vi "NI9188 Producer (Testing).vi"(5 "TDMS File Path":path, 7 "Logging Mode":i32(ring)=10231 items=["Off"=10231, "Log and Read"=15842], 8 "error in":errorcluster, 9 "Samples per Channel":i32=100, 10 "Sample Rate":dbl=100000.0, 11 "Data Queue":refnum<queue>) -> (0 "error out":errorcluster, 2 "Restart":bool)   [LabVIEW 2013]
uses:
  <vilib>/DAQmx/create/channels.llb/DAQmx Create Channel (AI-Voltage-Basic).vi
  <vilib>/DAQmx/configure/timing.llb/DAQmx Timing (Sample Clock).vi
  <vilib>/DAQmx/configure/task.llb/DAQmx Configure Logging (TDMS).vi
  <vilib>/DAQmx/create/channels.llb/DAQmx Create Channel (CO-Pulse Generation-Frequency).vi
  <vilib>/DAQmx/configure/timing.llb/DAQmx Timing (Implicit).vi
  <vilib>/DAQmx/configure/trigger.llb/DAQmx Start Trigger (Digital Edge).vi
  SCM Breakdown Locator/UDP Heartbeat Globals.vi
  Execution Control Global.vi
  <vilib>/DAQmx/read.llb/DAQmx Read (Analog 1D Wfm NChan NSamp).vi
  <resource>/objmgr/daqmx.rc
panel:
  out "name":string
  in  "Remote UDP Port":u16=31416
  out "Spark Flag Synch\nLoop Time (ms)":u32
  in  "Stop":bool
  out "Spark!":bool
  in  "Local UDP Port":u16=31417
  in  "Synch Delay (ms)":u16=50
  out "ms since last read":u32
  out "Waveform Graph":waveform(dbl)[](graph)
  out "Actual Sample Rate":dbl=1000.0 format="%0.2f"
  # "Acquired Data"
  # "Settings"
  # "Logging Settings"
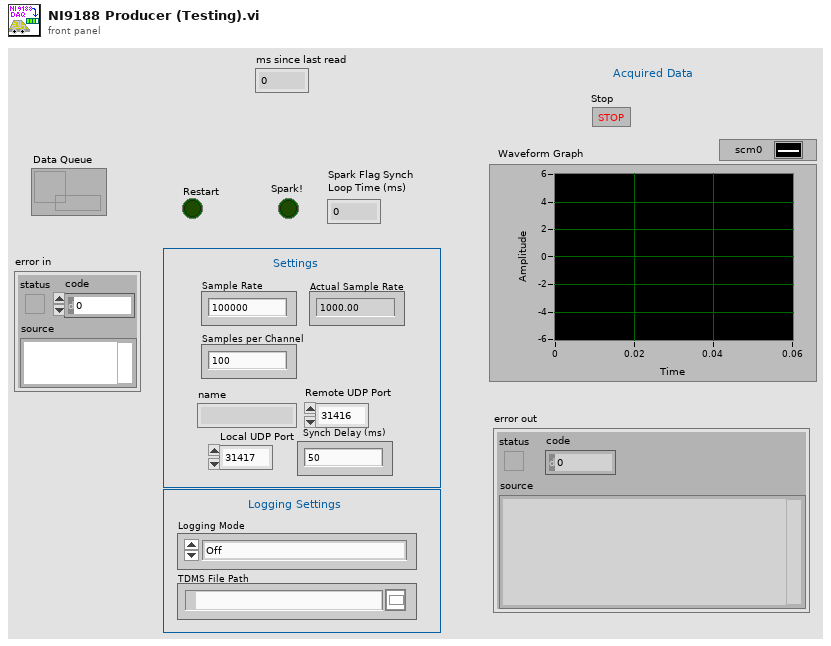
[diagram p1: front panel]
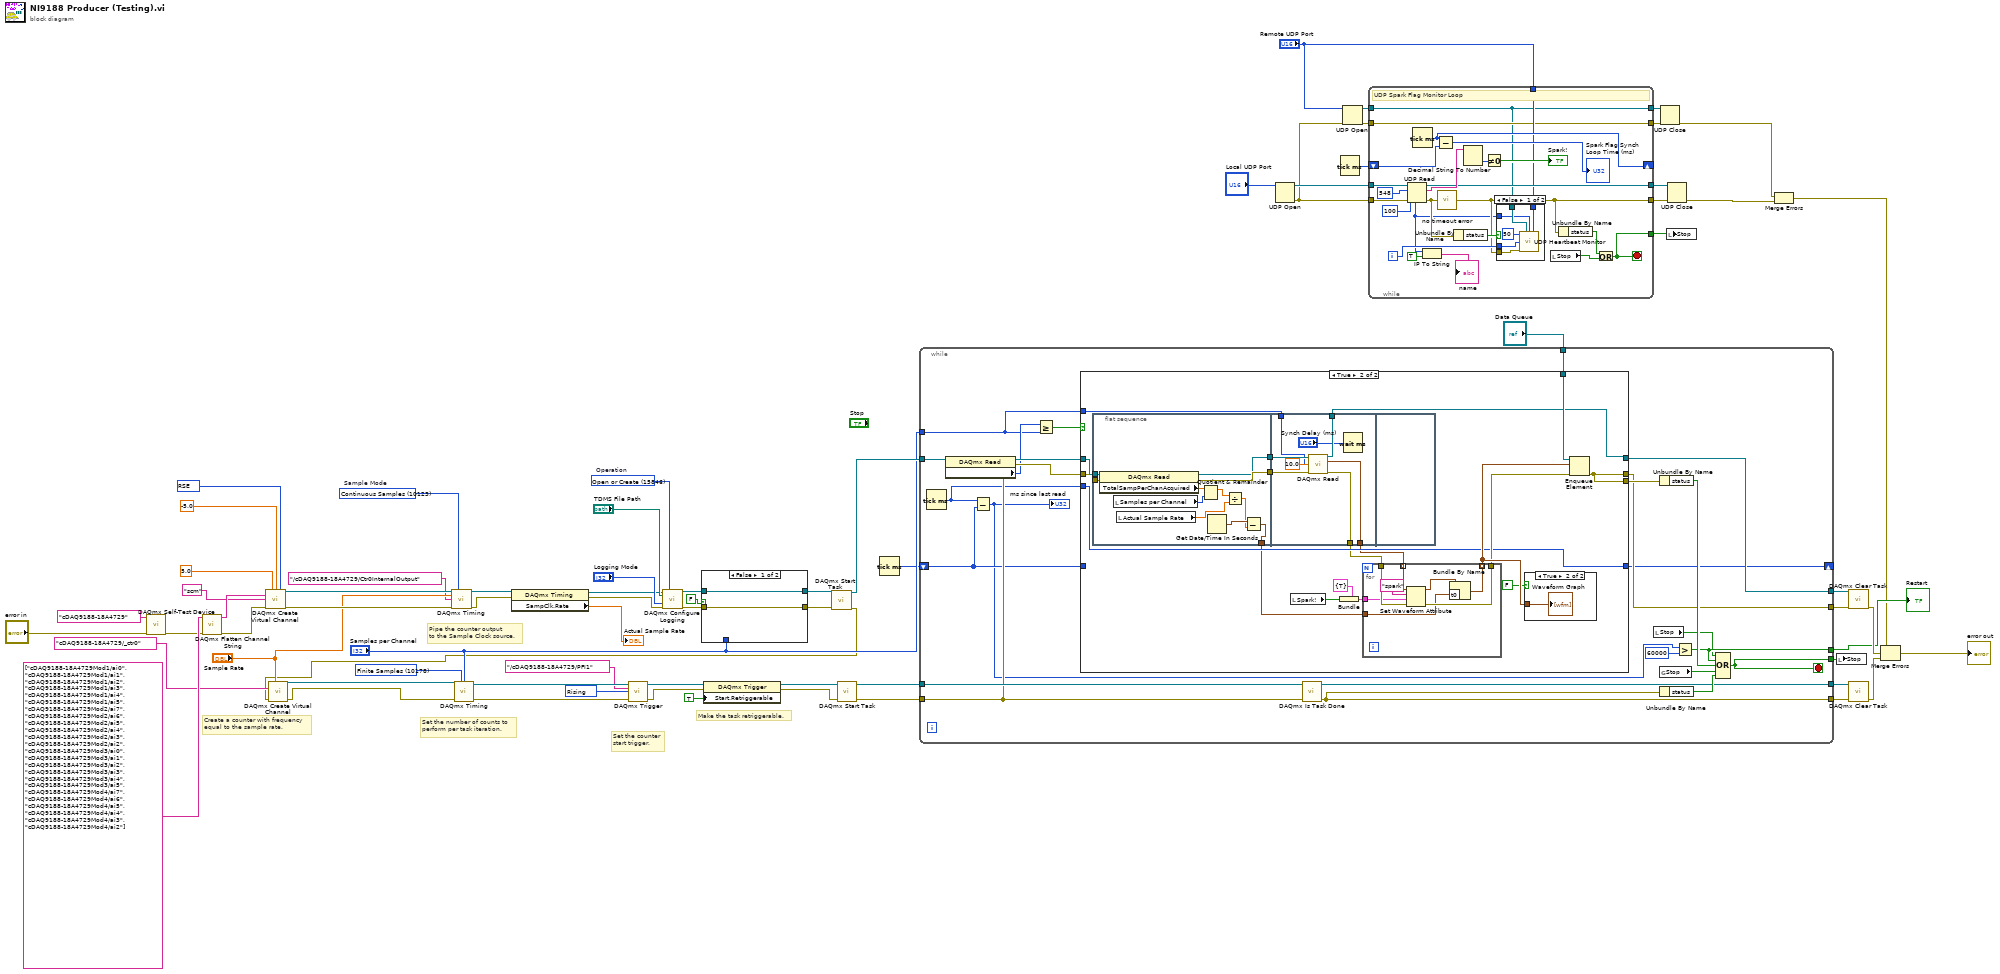
[diagram p0: block diagram]
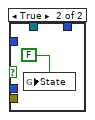
[diagram p2: hidden frame]
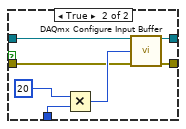
[diagram p3: hidden frame]
diagram:
  w30 = 10280 items=["Rising"=10280, "Falling"=10171] ("edge")
  w64 = 10083 items=["default"=-1, "RSE"=10083, "NRSE"=10078, "Differential"=10106, "Pseudodifferential"=12529] ("Terminal Configuration")
  w54 = 10178 items=["Finite Samples"=10178, "Continuous Samples"=10123, "Hardware Timed Single Point"=12522] ("sample mode")
  w67 = 15846 items=["Open"=10437, "Open or Create"=15846, "Create or Replace"=15847, "Create"=15848]  # Operation
  w70 = 10123 items=["Finite Samples"=10178, "Continuous Samples"=10123, "Hardware Timed Single Point"=12522]  # Sample Mode
  # "Set the counter\nstart trigger."
  # "Make the task retriggerable."
  # "Set the number of counts to\nperform per task iteration."
  # "Pipe the counter output\nto the Sample Clock source."
  # "Create a counter with frequency\nequal to the sample rate."
  n1 = call <vilib>:"DAQmx Self-Test Device.vi"("device in"=tag "cDAQ9188-18A4729", "error in"="error in") -> ("error out"=w21:errorcluster)  [unwired: 13 in]
  n2 = call <vilib>:"DAQmx Flatten Channel String.vi"("names in"=tag[] ["cDAQ9188-18A4729Mod1/ai0", "cDAQ9188-18A4729Mod1/ai1", "cDAQ9188-18A4729Mod1/ai2", "cDAQ9188-18A4729Mod1/ai3", "cDAQ9188-18A4729Mod1/ai4", "cDAQ9188-18A4729Mod1/ai5", "cDAQ9188-18A4729Mod2/ai7", "cDAQ9188-18A4729Mod2/ai6", "cDAQ9188-18A4729Mod2/ai5", "cDAQ9188-18A4729Mod2/ai4", "cDAQ9188-18A4729Mod2/ai3", "cDAQ9188-18A4729Mod2/ai2", "cDAQ9188-18A4729Mod3/ai0", "cDAQ9188-18A4729Mod3/ai1", "cDAQ9188-18A4729Mod3/ai2", "cDAQ9188-18A4729Mod3/ai3", "cDAQ9188-18A4729Mod3/ai4", "cDAQ9188-18A4729Mod3/ai5", "cDAQ9188-18A4729Mod4/ai7", "cDAQ9188-18A4729Mod4/ai6", "cDAQ9188-18A4729Mod4/ai5", "cDAQ9188-18A4729Mod4/ai4", "cDAQ9188-18A4729Mod4/ai3", "cDAQ9188-18A4729Mod4/ai2"], "error in"=w21) -> ("names out"=w60:string, "error out"=w59:errorcluster)  [unwired: 12 in]
  n3 = call-poly <vilib>:"DAQmx Create Virtual Channel.vi"("maximum value"=5.0 ("Max Voltage"), "minimum value"=-5.0 ("Min Voltage"), "input terminal configuration"=w64, "physical channels"=w60, "name to assign"="scm", "error in"=w59) -> ("task out"=w68:refnum<k21>, "error out"=w69:errorcluster)  [unwired: 8 in]
  n4 = call-poly <vilib>:"DAQmx Timing.vi"("task/channels in"=w68, "sample mode"=w70, "rate"="Sample Rate", "source"=tag "/cDAQ9188-18A4729/Ctr0InternalOutput" ("CO.Pulse.Term"), "error in"=w69) -> ("task out"=w72:refnum<k21>, "error out"=w71:errorcluster)  [unwired: 9 in]
  n5 = property class="DAQmx Timing"(reference=w72, error in=w71) -> (reference out=w34:refnum<k21>, error out=w33:errorcluster, "SampClk.Rate"=→"Actual Sample Rate":dbl)
  n6 = call-poly <vilib>:"DAQmx Configure Logging.vi"("task/channels in"=w34, "operation"=w67, "file path"="TDMS File Path", "logging mode"="Logging Mode", "error in"=w33) -> ("task out"=w39:refnum<k21>, "error out"=w38:errorcluster)  [unwired: 9 in]
  n7 = case shown="False" FALSE {
    tunnel: w39 -> [w74 w80]
    tunnel: w38 -> [w73 w79]
    tunnel: [w74 w78] -> w37
    tunnel: [w73 w77] -> w36
    tunnel: "Samples per Channel" -> [_ w75]
    frame False {
    }
    frame True {
      n8 = Multiply(x=u32 20, y=w75) -> (x*y=w81:u32)
      n9 = call <vilib>:"DAQmx Configure Input Buffer.vi"("task/channels in"=w80, "buffer size (in samples per channel)"=w81, "error in"=w79) -> ("task out"=w78:refnum<k21>, "error out"=w77:errorcluster)  [unwired: 11 in]
    }
  }
  n10 = call <vilib>:"DAQmx Start Task.vi"("task/channels in"=w37, "error in"=w36) -> ("task out"=w46:refnum<k21>, "error out"=w25:errorcluster)  [unwired: 12 in]
  n11 = call-poly <vilib>:"DAQmx Create Virtual Channel.vi"("frequency"="Sample Rate", "counter"=tag "cDAQ9188-18A4729/_ctr0" ("Counter*"), "error in"=w25) -> ("task out"=w27:refnum<k21>, "error out"=w26:errorcluster)  [unwired: 11 in]
  n12 = call-poly <vilib>:"DAQmx Timing.vi"("task/channels in"=w27, "sample mode"=w54, "samples per channel"="Samples per Channel", "error in"=w26) -> ("task out"=w52:refnum<k21>, "error out"=w51:errorcluster)  [unwired: 10 in]
  n13 = call-poly <vilib>:"DAQmx Trigger.vi"("task/channels in"=w52, "source"=tag "/cDAQ9188-18A4729/PFI1" ("Trigger Source"), "edge"=w30, "error in"=w51) -> ("task out"=w50:refnum<k21>, "error out"=w49:errorcluster)  [unwired: 10 in]
  n14 = property class="DAQmx Trigger"(reference=w50, error in=w49, "Start.Retriggerable"=TRUE) -> (reference out=w45:refnum<k21>, error out=w44:errorcluster)
  n15 = call <vilib>:"DAQmx Start Task.vi"("task/channels in"=w45, "error in"=w44) -> ("task out"=w43:refnum<k21>, "error out"=w42:errorcluster)  [unwired: 12 in]
  n16 = Tick Count (ms)() -> (millisecond timer value=w24:u32)
  n17 = while {
    tunnel: "Samples per Channel" -> [w84]
    tunnel: w46 -> [w97]
    tunnel: [w102] -> w56
    tunnel: [w101] -> w55
    tunnel: w43 -> [w104]
    tunnel: w42 -> [w94]
    tunnel: [w100] -> w41
    tunnel: [w99] -> w40
    tunnel: "Data Queue" -> [w91]
    shift-right: [w88] -> _
    shift-left: w24 -> [w90]
    tunnel: [w86] -> w19
    tunnel: [w82] -> w11
    stop <- w82 stop-if-true
    n18 = Tick Count (ms)() -> (millisecond timer value=w89:u32)
    n19 = property class="DAQmx Read"(reference=w97, error in=w94) -> (reference out=w96:refnum<k21>, error out=w95:errorcluster, "Status:Available Samples Per Channel"=w92:u32)
    n20 = Subtract(x=w89, y=w90) -> (x-y=w85:u32)
    "ms since last read" <- w85
    n21 = Greater Or Equal?(x=w92, y=w84) -> (x >= y?=w93:bool)
    n22 = case shown="True" w93 {
      tunnel: [w107 w124] -> w105
      tunnel: w96 -> [w108 w127]
      tunnel: w95 -> [w107 w126]
      tunnel: [w108 w111] -> w102
      tunnel: [w107 w124] -> w101
      tunnel: w91 -> [_ w125]
      tunnel: [w109 w121] -> w88
      tunnel: w90 -> [w109 _]
      tunnel: w89 -> [_ w121]
      tunnel: w84 -> [_ w115]
      frame False {
      }
      frame True {
        n23 = flat-sequence {
          tunnel: w126 -> [w137]
          tunnel: w127 -> [w138]
          tunnel: [w135] -> w117
          tunnel: [w136] -> w116
          tunnel: [w133] -> w114
          tunnel: w117 -> [w146]
          tunnel: w116 -> [w145]
          tunnel: w115 -> [w143]
          tunnel: [w142] -> w113
          tunnel: [w141] -> w112
          tunnel: [w140] -> w111
          frame #0 {
            n24 = property class="DAQmx Read"(reference=w138, error in=w137) -> (reference out=w135:refnum<k21>, error out=w136:errorcluster, "TotalSampPerChanAcquired"=w131:dbl)
            n25 = local read "Samples per Channel"() -> (w132:i32)
            n26 = local read "Actual Sample Rate"() -> (w129:dbl)
            n27 = Quotient & Remainder(x=w131, y=w132) -> (x-y*floor(x/y)=w130:dbl)  [unwired: 1 out]
            n28 = Get Date/Time In Seconds() -> (seconds since 1Jan1904=w134:timestamp)
            n29 = Divide(x=w130, y=w129) -> (x/y=w128:dbl)
            n30 = Subtract(x=w134, y=w128) -> (x-y=w133:timestamp)
          }
          frame #1 {
            n31 = call-poly <vilib>:"DAQmx Read.vi"("task/channels in"=w146, "number of samples per channel"=w143, "timeout"=10.0, "error in"=w145) -> ("task out"=w140:refnum<k21>, "data"=w141:waveform(dbl)[], "error out"=w142:errorcluster)  [unwired: 9 in]
            n32 = Wait (ms)(milliseconds to wait="Synch Delay (ms)") -> ()  [unwired: 1 out]
          }
          frame #2 {
          }
        }
        n33 = local read "Spark!"() -> (w110:bool)
        n34 = Bundle(cluster=cluster{bool} {TRUE} ("value"), w110) -> (w118:cluster{bool})
        n35 = for {
          tunnel: w112 -> [w154] mode=indexing
          tunnel: [w148] -> w123 mode=indexing
          tunnel: w113 -> [w153]
          tunnel: [w152] -> w122
          tunnel: w118 -> [w150]
          tunnel: w114 -> [w147]
          n36 = Set Waveform Attribute(4:w153, 5:w150, 6:"spark" ("name"), 7:w154) -> (0:w152:errorcluster, 3:w149:waveform(dbl))  [unwired: 1 out]
          n37 = Bundle By Name(cluster=w149, "t0"=w147) -> (w148:waveform(dbl))
        }
        n38 = case shown="True" FALSE {
          tunnel: w123 -> [_ w155]
          frame False {
          }
          frame True {
            "Waveform Graph" <- w155
          }
        }
        n39 = Enqueue Element(queue=w125, element=w123, error in (no error)=w122) -> (error out=w124:errorcluster)  [unwired: 1 in, 2 out]
      }
    }
    n40 = call <vilib>:"DAQmx Is Task Done.vi"("task/channels in"=w104, "error in"=w94) -> ("task out"=w100:refnum<k21>, "error out"=w99:errorcluster)  [unwired: 11 in, 1 out]
    n41 = local read "Stop"() -> (w83:bool)
    n42 = Unbundle By Name(w105) -> ("status"=w106:bool)
    n43 = Unbundle By Name(w99) -> ("status"=w103:bool)
    n44 = global read "Execution Control Global.vi" "Stop"() -> (w98:bool)
    n45 = Greater?(x=w85, y=u32 60000) -> (0:w86:bool)
    n46 = Compound Arithmetic op=OR(w83, w86, w106, w98, w103) -> (w82:bool)
  }
  "Restart" <- w19
  n47 = UDP Open(11:"Local UDP Port") -> (port=w16:refnum<k16>, 0:w7:errorcluster)  [unwired: 4 in, 1 out]
  n48 = Tick Count (ms)() -> (millisecond timer value=w10:u32)
  n49 = UDP Open(8:w7, 11:"Remote UDP Port") -> (port=w8:refnum<k16>, 0:w6:errorcluster)  [unwired: 3 in, 1 out]
  n50 = while {
    tunnel: w16 -> [w178]
    tunnel: w7 -> [w177]
    tunnel: [w163] -> w15
    tunnel: [w162] -> w14
    tunnel: [w173] -> w12
    shift-right: [w168] -> _
    shift-left: w10 -> [w170]
    tunnel: "Remote UDP Port" -> [w161]
    tunnel: w8 -> [w159]
    tunnel: [w160] -> w5
    tunnel: w6 -> [w160]
    tunnel: [w159] -> w4
    i -> [w165]
    stop <- w173 stop-if-true
    # "UDP Spark Flag Monitor Loop"
    n51 = UDP Read(connection ID=w178, max size (548)=548 ("max bytes/read"), timeout ms (25000)=100, 8:w177) -> (data out=w179:string, error out=w166:errorcluster, 3:w162:refnum<k16>, 6:w158:u32)  [unwired: 1 out]
    n52 = Tick Count (ms)() -> (millisecond timer value=w168:u32)
    n53 = IP To String(1:TRUE ("dot notation? (F)"), 2:w158) -> (0:→"name":string)
    n54 = Subtract(x=w168, y=w170) -> (x-y=→"Spark Flag Synch\nLoop Time (ms)":u32)
    n55 = call "no timeout error.vi"("error in (no error)"=w166) -> ("error out"=w163:errorcluster)
    n56 = Unbundle By Name(w166) -> ("status"=w164:bool)
    n57 = Decimal String To Number(string=w179) -> (number=w172:i32)  [unwired: 2 in, 1 out]
    n58 = Not Equal To 0?(x=w172) -> (x != 0?=→"Spark!":bool)
    n59 = case shown="False" w164 {
      tunnel: w165 -> [w184 _]
      tunnel: w163 -> [w183 _]
      tunnel: w159 -> [w182 _]
      tunnel: w161 -> [w181 _]
      tunnel: w158 -> [w180 _]
      frame False {
        n60 = call "UDP Heartbeat Monitor.vi"("Interval Length"=50, "connection ID"=w182, "Remote UDP Address"=w180, "Remote UDP Port"=w181, "Count"=w184, "error in (no error)"=w183) -> ()  [unwired: 9 in, 1 out]
      }
      frame True {
        n61 = global write "UDP Heartbeat Globals.vi" "State"(FALSE) -> ()
      }
    }
    n62 = local read "Stop"() -> (w174:bool)
    n63 = Unbundle By Name(w163) -> ("status"=w175:bool)
    n64 = Or(x=w175, y=w174) -> (x .or. y?=w173:bool)
  }
  n65 = UDP Close(connection ID=w4, 8:w5) -> (error out=w2:errorcluster)  [unwired: 1 out]
  n66 = local write "Stop"(w12) -> ()
  n67 = UDP Close(connection ID=w14, 8:w15) -> (error out=w1:errorcluster)  [unwired: 1 out]
  n68 = Merge Errors(w2, w1) -> (w3:errorcluster)
  n69 = local write "Stop"(w11) -> ()
  n70 = call <vilib>:"DAQmx Clear Task.vi"("task in"=w56, "error in"=w55) -> ("error out"=w28:errorcluster)  [unwired: 13 in]
  n71 = call <vilib>:"DAQmx Clear Task.vi"("task in"=w41, "error in"=w40) -> ("error out"=w29:errorcluster)  [unwired: 13 in]
  n72 = Merge Errors(w3, w28, w29) -> (→"error out":errorcluster)
